vi "DrawToolPosition.vi"(9 "Setup":T1, 10 "Y":dbl, 11 "X":dbl) -> (3 "blob":picture)   [LabVIEW 2023]
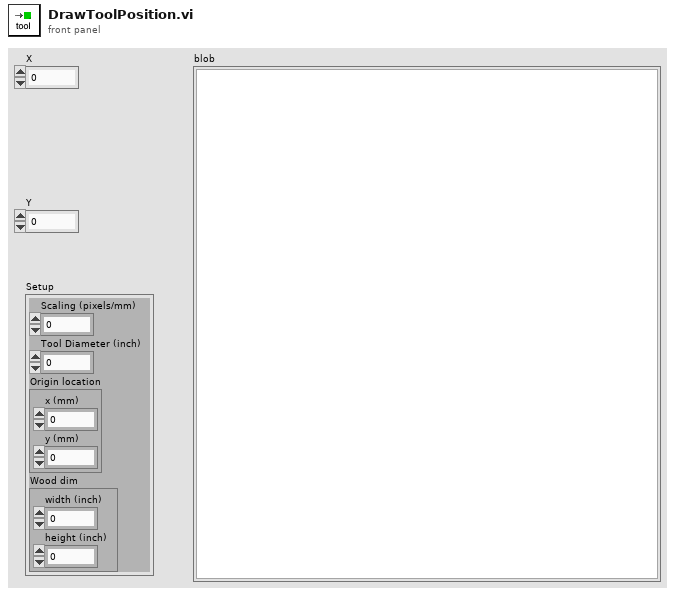
[diagram p1: front panel]
types:
  T1 = cluster{"Scaling (pixels/mm)":dbl, "Tool Diameter (inch)":dbl, "Origin location":cluster{"x (mm)":i16, "y (mm)":i16}, "Wood dim":cluster{"width (inch)":dbl, "height (inch)":dbl}}
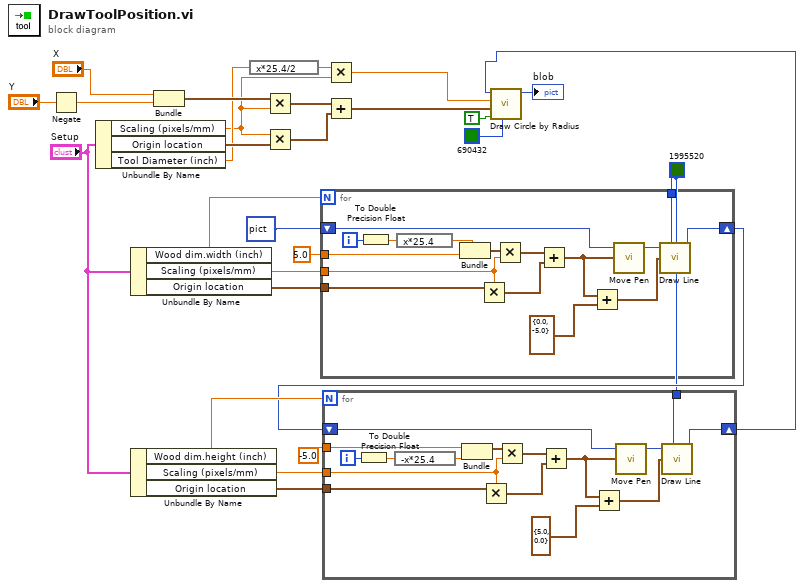
[diagram p0: block diagram]
diagram:
  w1 = u32 1995520 ("color(black)")
  n1 = Negate(x="Y") -> (-x=w16:dbl)
  n2 = Unbundle By Name("Setup") -> ("Scaling (pixels/mm)"=w15:dbl, "Origin location"=w24:cluster{"x (mm)":i16, "y (mm)":i16}, "Tool Diameter (inch)"=w20:dbl)
  n3 = Unbundle By Name("Setup") -> ("Wood dim.width (inch)"=w9:dbl, "Scaling (pixels/mm)"=w13:dbl, "Origin location"=w12:cluster{"x (mm)":i16, "y (mm)":i16})
  n4 = Unbundle By Name("Setup") -> ("Wood dim.height (inch)"=w8:dbl, "Scaling (pixels/mm)"=w6:dbl, "Origin location"=w7:cluster{"x (mm)":i16, "y (mm)":i16})
  n5 = Bundle("X"="X", w16) -> (w27:cluster{"X":dbl, dbl})  [unwired: 1 in]
  n6 = expression code="x*25.4/2"(w20) -> (w26:dbl)
  n7 = Multiply(x=w27, y=w15) -> (x*y=w23:cluster{"X":dbl, dbl})
  n8 = Multiply(x=w15, y=w24) -> (x*y=w25:cluster{"x (mm)":dbl, "y (mm)":dbl})
  n9 = for {
    N: w9 -> [_]
    tunnel: 5.0 -> [w41]
    tunnel: w13 -> [w38]
    tunnel: w12 -> [w39]
    shift-right: [w33] -> w3
    shift-left: picture data[5B] ("picture") -> [w34]
    tunnel: w1 -> [w29]
    i -> [w32]
    n10 = To Double Precision Float(number=w32) -> (double precision float=w30:dbl)
    n11 = expression code="x*25.4"(w30) -> (w31:dbl)
    n12 = Bundle(w31, w41) -> (w40:cluster{dbl, dbl})  [unwired: 1 in]
    n13 = Multiply(x=w39, y=w38) -> (x*y=w42:cluster{"x (mm)":dbl, "y (mm)":dbl})
    n14 = Multiply(x=w40, y=w38) -> (x*y=w43:cluster{dbl, dbl})
    n15 = Add(x=w43, y=w42) -> (x+y=w37:cluster{dbl, dbl})
    n16 = Add(x=w37, y=cluster{dbl, dbl} {0.0, -5.0}) -> (x+y=w35:cluster{dbl, dbl})
    n17 = call <vilib>:"Move Pen.vi"("new position"=w37, "picture"=w34) -> ("new picture"=w44:picture)  [unwired: 3 in]
    n18 = call <vilib>:"Draw Line.vi"("picture"=w44, "end point"=w35, "color(black)"=w29) -> ("new picture"=w33:picture)  [unwired: 6 in]
  }
  n19 = for {
    N: w8 -> [_]
    tunnel: w6 -> [w56]
    tunnel: w7 -> [w57]
    shift-right: [w51] -> w2
    shift-left: w3 -> [w52]
    tunnel: -5.0 -> [w47]
    tunnel: w1 -> [w45]
    i -> [w50]
    n20 = To Double Precision Float(number=w50) -> (double precision float=w49:dbl)
    n21 = expression code="-x*25.4"(w49) -> (w48:dbl)
    n22 = Bundle(w47, w48) -> (w46:cluster{dbl, dbl})  [unwired: 1 in]
    n23 = Multiply(x=w57, y=w56) -> (x*y=w58:cluster{"x (mm)":dbl, "y (mm)":dbl})
    n24 = Multiply(x=w46, y=w56) -> (x*y=w59:cluster{dbl, dbl})
    n25 = Add(x=w59, y=w58) -> (x+y=w55:cluster{dbl, dbl})
    n26 = Add(x=w55, y=cluster{dbl, dbl} {5.0, 0.0}) -> (x+y=w53:cluster{dbl, dbl})
    n27 = call <vilib>:"Move Pen.vi"("new position"=w55, "picture"=w52) -> ("new picture"=w60:picture)  [unwired: 3 in]
    n28 = call <vilib>:"Draw Line.vi"("picture"=w60, "end point"=w53, "color(black)"=w45) -> ("new picture"=w51:picture)  [unwired: 6 in]
  }
  n29 = Multiply(x=w26, y=w15) -> (x*y=w28:dbl)
  n30 = Add(x=w23, y=w25) -> (x+y=w19:cluster{dbl, dbl})
  n31 = call <vilib>:"Draw Circle by Radius.vi"("color(black)"=u32 690432, "fill?(F)"=TRUE, "pixel center"=w19, "radius"=w28, "picture"=w2) -> ("new picture"=→"blob":picture)  [unwired: 6 in]
